vi "FPGA-Start-15-07-17.vi"() -> (0 "error out":errorcluster, 1 "FPGA VI Reference Out":refnum<k20>)   [LabVIEW 2017]
uses:
  <vilib>/rvi/interface/nirviOpenFPGA/nirviOpenFPGA.xnode
  <vilib>/rvi/interface/nirviMethod/nirviMethod.xnode
  <vilib>/LabVIEW Targets/FPGA/cRIO/shared/nicrio_ModuleControls/nicrio_cRIO-9871_FlowControlEnum.ctl
  <vilib>/LabVIEW Targets/FPGA/cRIO/shared/nicrio_ModuleControls/nicrio_cRIO-9871_StopBitsEnum.ctl
  <vilib>/LabVIEW Targets/FPGA/cRIO/shared/nicrio_ModuleControls/nicrio_cRIO-9871_ParityEnum.ctl
  <vilib>/LabVIEW Targets/FPGA/cRIO/shared/nicrio_ModuleControls/nicrio_cRIO-9871_DataBitsEnum.ctl
  <vilib>/LabVIEW Targets/FPGA/cRIO/shared/nicrio_ModuleControls/nicrio_cRIO-9871_BaudRateEnum.ctl
  <vilib>/rvi/interface/nirviReadWriteControl/nirviReadWriteControl.xnode
  FPGA/FPGA-Programm-05-17.vi
  <vilib>/FPGAPlugInAG/cRIO-9114/niLvFpga_ReadFifo_cRIO-9114.vi
  <vilib>/rvi/errors/niLvFpgaMergeErrorWithErrorCode.vi
  FPGA Bitfiles/HAGAR-V_FPGATarget_FPGA-Programm-05_gdVwCsZS6sg.lvbitx
  <vilib>/FPGAPlugInAG/cRIO-9114/niLvFpga_Open_cRIO-9114.vi
  <vilib>/FPGAPlugInAG/cRIO-9114/niLvFpga_Reset_cRIO-9114.vi
  NiFpgaLv.dll
  <vilib>/Utility/error.llb/Error Cluster From Error Code.vi
  <vilib>/rvi/errors/niLvFpgaAdjustHostInterfaceError.vi
  <vilib>/FPGAPlugInAG/cRIO-9114/niLvFpga_Run_cRIO-9114.vi
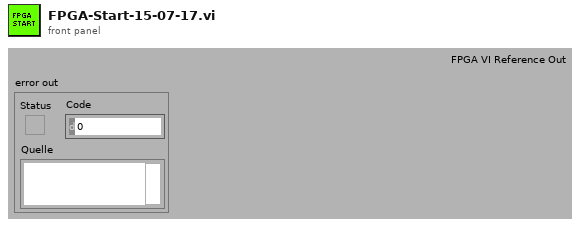
[diagram p1: front panel]
types:
  T1 = cluster{"H1-Valve2":u32, "H1-Spare2":u32, "H1-Spare1":u32, "H1-Valve1":u32, "H0-Drier":u32, "HL-Licor":u32, "H2-ECD2":u32, "H2-Oven":u32, "H2-Spare1":u32, "H2-Col2":u32, "H2-Col1":u32, "H2-ECD1":u32, "H1-Inlet":u32}
  T2 = cluster{"H1-Valve2":bool, "H1-Spare2":bool, "H1-Spare1":bool, "H1-Valve1":bool, "H0-Drier":bool, "HL-Licor":bool, "H2-ECD2":bool, "H2-Oven":bool, "H2-Spare1":bool, "H2-Col2":bool, "H2-Col1":bool, "H2-ECD1":bool, "H1-Inlet":bool}
  T3 = cluster{"Mod6/DIO 0":bool, "Mod6/DIO 1":bool, "Mod6/DIO 2":bool, "Mod6/DIO 3":bool, "Mod6/DIO 4":bool, "Mod6/DIO 5":bool, "Mod6/DIO 6":bool, "Mod6/DIO 7":bool, "Mod6/DIO 8":bool, "Mod6/DIO 9":bool, "Mod6/DIO 10":bool, "Mod6/DIO 11":bool, "Mod6/DIO 12":bool, "Mod6/DIO 13":bool, "Mod6/DIO 14":bool, "Mod6/DIO 15":bool, "Mod6/DIO 16":bool, "Mod6/DIO 17":bool, "Mod6/DIO 18":bool, "Mod6/DIO 19":bool, "Mod6/DIO 20":bool, "Mod6/DIO 21":bool, "Mod6/DIO 22":bool, "Mod6/DIO 23":bool, "Mod6/DIO 24":bool, "Mod6/DIO 25":bool, "Mod6/DIO 26":bool, "Mod6/DIO 27":bool, "Mod6/DIO 28":bool, "Mod6/DIO 29":bool, "Mod6/DIO 30":bool, "Mod6/DIO 31":bool}
  T4 = cluster{"Mod5/DIO 0":bool, "Mod5/DIO 1":bool, "Mod5/DIO 2":bool, "Mod5/DIO 3":bool, "Mod5/DIO 4":bool, "Mod5/DIO 5":bool, "Mod5/DIO 6":bool, "Mod5/DIO 7":bool, "Mod5/DIO 8":bool, "Mod5/DIO 9":bool, "Mod5/DIO 10":bool, "Mod5/DIO 11":bool, "Mod5/DIO 12":bool, "Mod5/DIO 13":bool, "Mod5/DIO 14":bool, "Mod5/DIO 15":bool, "Mod5/DIO 16":bool, "Mod5/DIO 17":bool, "Mod5/DIO 18":bool, "Mod5/DIO 19":bool, "Mod5/DIO 20":bool, "Mod5/DIO 21":bool, "Mod5/DIO 22":bool, "Mod5/DIO 23":bool, "Mod5/DIO 24":bool, "Mod5/DIO 25":bool, "Mod5/DIO 26":bool, "Mod5/DIO 27":bool, "Mod5/DIO 28":bool, "Mod5/DIO 29":bool, "Mod5/DIO 30":bool, "Mod5/DIO 31":bool}
  T5 = typedef "nicrio_cRIO-9871_BaudRateEnum.ctl" = enum16{"75 bps", "110 bps", "134 bps", "150 bps", "300 bps", "600 bps", "1200 bps", "1800 bps", "2400 bps", "4800 bps", "7200 bps", "9600 bps", "14.4 kbps", "19.2 kbps", "28.8 kbps", "38.4 kbps", "57.6 kbps", "115.2 kbps", "230.4 kbps", "460.8 kbps", "921.6 kbps"}
  T6 = typedef "nicrio_cRIO-9871_DataBitsEnum.ctl" = enum8{"5", "6", "7", "8"}
  T7 = typedef "nicrio_cRIO-9871_ParityEnum.ctl" = enum8{"None", "Odd", "Even", "Mark", "Space"}
  T8 = typedef "nicrio_cRIO-9871_StopBitsEnum.ctl" = enum8{"1", "1.5", "2"}
  T9 = typedef "nicrio_cRIO-9871_FlowControlEnum.ctl" = enum8{"None", "Software (XON / XOFF)", "Hardware (RTS / CTS)"}
  T10 = cluster{"Mod7/Port1":cluster{"Baud Rate":T5, "Data Bits":T6, "Parity":T7, "Stop Bits":T8, "Flow Control":T9}, "Mod7/Port2":cluster{"Baud Rate":T5, "Data Bits":T6, "Parity":T7, "Stop Bits":T8, "Flow Control":T9}, "Mod7/Port3":cluster{"Baud Rate":T5, "Data Bits":T6, "Parity":T7, "Stop Bits":T8, "Flow Control":T9}, "Mod7/Port4":cluster{"Baud Rate":T5, "Data Bits":T6, "Parity":T7, "Stop Bits":T8, "Flow Control":T9}, "Mod8/Port1":cluster{"Baud Rate":T5, "Data Bits":T6, "Parity":T7, "Stop Bits":T8, "Flow Control":T9}, "Mod8/Port2":cluster{"Baud Rate":T5, "Data Bits":T6, "Parity":T7, "Stop Bits":T8, "Flow Control":T9}, "Mod8/Port3":cluster{"Baud Rate":T5, "Data Bits":T6, "Parity":T7, "Stop Bits":T8, "Flow Control":T9}, "Mod8/Port4":cluster{"Baud Rate":T5, "Data Bits":T6, "Parity":T7, "Stop Bits":T8, "Flow Control":T9}}
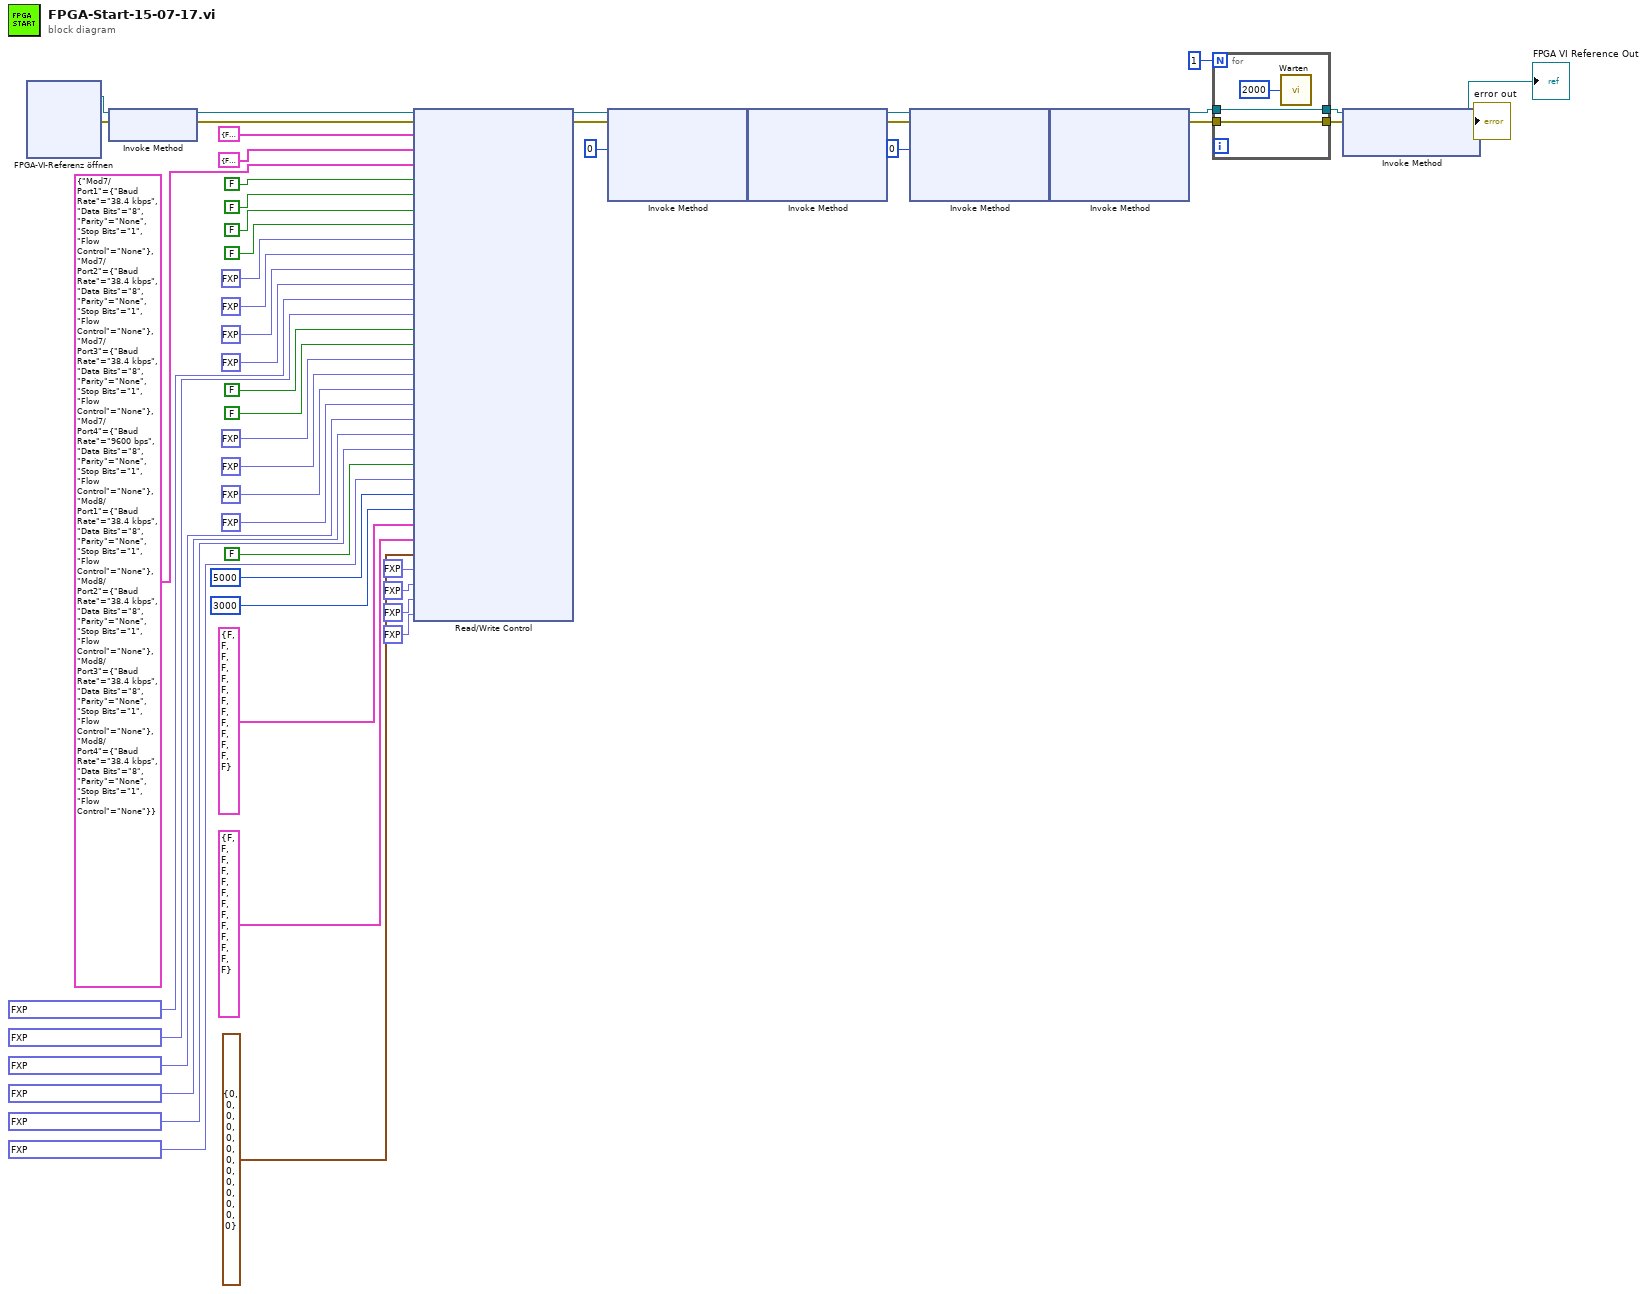
[diagram p0: block diagram]
diagram:
  n1 = xnode "FPGA-VI-Referenz öffnen"() -> ("FPGA-VI-Referenz (Ausgang)"=w33:refnum<k20>, "Fehler (Ausgang)"=w32:errorcluster)  [unwired: 2 in]
  n2 = xnode "Invoke Method"("FPGA-VI-Referenz (Eingang)"=w33, "Fehler (Eingang)"=w32) -> ("FPGA-VI-Referenz (Ausgang)"=w51:refnum<k20>, "Fehler (Ausgang)"=w52:errorcluster)
  n3 = xnode "Read/Write Control"("FPGA-VI-Referenz (Eingang)"=w51, "Fehler (Eingang)"=w52, "Mod5/DIOs"=T4 {"Mod5/DIO 0"=FALSE, "Mod5/DIO 1"=FALSE, "Mod5/DIO 2"=FALSE, "Mod5/DIO 3"=FALSE, "Mod5/DIO 4"=FALSE, "Mod5/DIO 5"=FALSE, "Mod5/DIO 6"=FALSE, "Mod5/DIO 7"=FALSE, "Mod5/DIO 8"=FALSE, "Mod5/DIO 9"=FALSE, "Mod5/DIO 10"=FALSE, "Mod5/DIO 11"=FALSE, "Mod5/DIO 12"=FALSE, "Mod5/DIO 13"=FALSE, "Mod5/DIO 14"=FALSE, "Mod5/DIO 15"=FALSE, "Mod5/DIO 16"=FALSE, "Mod5/DIO 17"=FALSE, "Mod5/DIO 18"=FALSE, "Mod5/DIO 19"=FALSE, "Mod5/DIO 20"=FALSE, "Mod5/DIO 21"=FALSE, "Mod5/DIO 22"=FALSE, "Mod5/DIO 23"=FALSE, "Mod5/DIO 24"=FALSE, "Mod5/DIO 25"=FALSE, "Mod5/DIO 26"=FALSE, "Mod5/DIO 27"=FALSE, "Mod5/DIO 28"=FALSE, "Mod5/DIO 29"=FALSE, "Mod5/DIO 30"=FALSE, "Mod5/DIO 31"=FALSE} ("Mod5/DIO"), "Mod6/DIOs"=T3 {"Mod6/DIO 0"=FALSE, "Mod6/DIO 1"=FALSE, "Mod6/DIO 2"=FALSE, "Mod6/DIO 3"=FALSE, "Mod6/DIO 4"=FALSE, "Mod6/DIO 5"=FALSE, "Mod6/DIO 6"=FALSE, "Mod6/DIO 7"=FALSE, "Mod6/DIO 8"=FALSE, "Mod6/DIO 9"=FALSE, "Mod6/DIO 10"=FALSE, "Mod6/DIO 11"=FALSE, "Mod6/DIO 12"=FALSE, "Mod6/DIO 13"=FALSE, "Mod6/DIO 14"=FALSE, "Mod6/DIO 15"=FALSE, "Mod6/DIO 16"=FALSE, "Mod6/DIO 17"=FALSE, "Mod6/DIO 18"=FALSE, "Mod6/DIO 19"=FALSE, "Mod6/DIO 20"=FALSE, "Mod6/DIO 21"=FALSE, "Mod6/DIO 22"=FALSE, "Mod6/DIO 23"=FALSE, "Mod6/DIO 24"=FALSE, "Mod6/DIO 25"=FALSE, "Mod6/DIO 26"=FALSE, "Mod6/DIO 27"=FALSE, "Mod6/DIO 28"=FALSE, "Mod6/DIO 29"=FALSE, "Mod6/DIO 30"=FALSE, "Mod6/DIO 31"=FALSE} ("Mod6/DIO"), "KonfigSeriell"=T10 {"Mod7/Port1"={"Baud Rate"=enum."38.4 kbps", "Data Bits"=enum."8", "Parity"=enum."None", "Stop Bits"=enum."1", "Flow Control"=enum."None"}, "Mod7/Port2"={"Baud Rate"=enum."38.4 kbps", "Data Bits"=enum."8", "Parity"=enum."None", "Stop Bits"=enum."1", "Flow Control"=enum."None"}, "Mod7/Port3"={"Baud Rate"=enum."38.4 kbps", "Data Bits"=enum."8", "Parity"=enum."None", "Stop Bits"=enum."1", "Flow Control"=enum."None"}, "Mod7/Port4"={"Baud Rate"=enum."9600 bps", "Data Bits"=enum."8", "Parity"=enum."None", "Stop Bits"=enum."1", "Flow Control"=enum."None"}, "Mod8/Port1"={"Baud Rate"=enum."38.4 kbps", "Data Bits"=enum."8", "Parity"=enum."None", "Stop Bits"=enum."1", "Flow Control"=enum."None"}, "Mod8/Port2"={"Baud Rate"=enum."38.4 kbps", "Data Bits"=enum."8", "Parity"=enum."None", "Stop Bits"=enum."1", "Flow Control"=enum."None"}, "Mod8/Port3"={"Baud Rate"=enum."38.4 kbps", "Data Bits"=enum."8", "Parity"=enum."None", "Stop Bits"=enum."1", "Flow Control"=enum."None"}, "Mod8/Port4"={"Baud Rate"=enum."38.4 kbps", "Data Bits"=enum."8", "Parity"=enum."None", "Stop Bits"=enum."1", "Flow Control"=enum."None"}}, "FIFO leer"=FALSE, "Heizen?Trap1"=FALSE, "Heizen?PreMach1"=FALSE, "Heizen?PreMach2"=FALSE, "d0PreMach1"=fxp<+/-,18,18> 0.0, "d1PreMach1"=fxp<+/-,21,21> 1.0, "d0PreMach2"=fxp<+/-,18,18> 0.0, "d1PreMach2"=fxp<+/-,21,21> 1.0, "USetp[V]PreMach1"=fxp<+/-,26,5> 0.0, "USetp[V]PreMach2"=fxp<+/-,26,5> 0.0, "Heizen?MainMach1"=FALSE, "Heizen?MainMach2"=FALSE, "d0MainMach1"=fxp<+/-,18,18> 0.0, "d1MainMach1"=fxp<+/-,21,21> 1.0, "d0MainMach2"=fxp<+/-,18,18> 0.0, "d1MainMach2"=fxp<+/-,21,21> 1.0, "USetp[V]MainMach1"=fxp<+/-,26,5> 0.0, "USetp[V]MainMach2"=fxp<+/-,26,5> 0.0, "SetpointTrap1"=fxp<+/-,26,5> 0.0, "Heizen?Trap2"=FALSE, "SetpointTrap2"=fxp<+/-,26,5> 0.0, "Warten(us)"=u16 5000, "vor der Messung [us]Mach"=u16 3000, "LHHeizen1?"=T2 {"H1-Valve2"=FALSE, "H1-Spare2"=FALSE, "H1-Spare1"=FALSE, "H1-Valve1"=FALSE, "H0-Drier"=FALSE, "HL-Licor"=FALSE, "H2-ECD2"=FALSE, "H2-Oven"=FALSE, "H2-Spare1"=FALSE, "H2-Col2"=FALSE, "H2-Col1"=FALSE, "H2-ECD1"=FALSE, "H1-Inlet"=FALSE}, "LHHeizen2?"=T2 {"H1-Valve2"=FALSE, "H1-Spare2"=FALSE, "H1-Spare1"=FALSE, "H1-Valve1"=FALSE, "H0-Drier"=FALSE, "HL-Licor"=FALSE, "H2-ECD2"=FALSE, "H2-Oven"=FALSE, "H2-Spare1"=FALSE, "H2-Col2"=FALSE, "H2-Col1"=FALSE, "H2-ECD1"=FALSE, "H1-Inlet"=FALSE}, "LHPulse(us)"=T1 {"H1-Valve2"=0, "H1-Spare2"=0, "H1-Spare1"=0, "H1-Valve1"=0, "H0-Drier"=0, "HL-Licor"=0, "H2-ECD2"=0, "H2-Oven"=0, "H2-Spare1"=0, "H2-Col2"=0, "H2-Col1"=0, "H2-ECD1"=0, "H1-Inlet"=0}, "d0Trap1"=fxp<+/-,18,18> 0.0, "d1Trap1"=fxp<+/-,21,21> 1.0, "d0Trap2"=fxp<+/-,18,18> 0.0, "d1Trap2"=fxp<+/-,21,21> 1.0) -> ("FPGA-VI-Referenz (Ausgang)"=w35:refnum<k20>, "Fehler (Ausgang)"=w34:errorcluster)
  n4 = xnode "Invoke Method"("FPGA-VI-Referenz (Eingang)"=w35, "Fehler (Eingang)"=w34, "Anzahl der Elemente"=u32 0 ("Number of Elements")) -> ("FPGA-VI-Referenz (Ausgang)"=w56:refnum<k20>, "Fehler (Ausgang)"=w53:errorcluster, "Verbleibende Elemente"=w55:u32)  [unwired: 1 in, 1 out]
  n5 = xnode "Invoke Method"("FPGA-VI-Referenz (Eingang)"=w56, "Fehler (Eingang)"=w53, "Anzahl der Elemente"=w55) -> ("FPGA-VI-Referenz (Ausgang)"=w49:refnum<k20>, "Fehler (Ausgang)"=w45:errorcluster)  [unwired: 1 in, 2 out]
  n6 = xnode "Invoke Method"("FPGA-VI-Referenz (Eingang)"=w49, "Fehler (Eingang)"=w45, "Anzahl der Elemente"=u32 0 ("Number of Elements")) -> ("FPGA-VI-Referenz (Ausgang)"=w47:refnum<k20>, "Fehler (Ausgang)"=w44:errorcluster, "Verbleibende Elemente"=w46:u32)  [unwired: 1 in, 1 out]
  n7 = xnode "Invoke Method"("FPGA-VI-Referenz (Eingang)"=w47, "Fehler (Eingang)"=w44, "Anzahl der Elemente"=w46) -> ("FPGA-VI-Referenz (Ausgang)"=w37:refnum<k20>, "Fehler (Ausgang)"=w36:errorcluster)  [unwired: 1 in, 2 out]
  n8 = for {
    N: 1 -> [_]
    tunnel: w37 -> [w59]
    tunnel: [w59] -> w41
    tunnel: w36 -> [w58]
    tunnel: [w58] -> w39
    n9 = call "Warten"("Count(mSec)"=u32 2000) -> ()  [unwired: 1 out]
  }
  n10 = xnode "Invoke Method"("FPGA-VI-Referenz (Eingang)"=w41, "Fehler (Eingang)"=w39) -> ("FPGA-VI-Referenz (Ausgang)"=→"FPGA VI Reference Out":refnum<k20>, "Fehler (Ausgang)"=→"error out":errorcluster)  [unwired: 1 in]
